vi "sorter.vi"() -> ()   [LabVIEW 2016]
uses:
  <vilib>/vision/NI_Vision_Development_Module.lvlib
panel:
  out "motor":bool
  out "green no.":dbl
  out "red no.":dbl
  out "?":dbl(graph)
  out "Sensor":bool
  in  "STOP":bool
  in  "START":bool
  in  "Stop (F)":bool
  out "?":dbl
  out "?":dbl
  out "green":bool
  out "red":bool
  out "?":dbl[](array[numeric]) format="%.2f"
  out "?":T1(plugin-control)
  # "Color Sorting Machine"
  # "Image Processing Indicators"
  # "Supervisory Control Panel"
  # "Motor Speed"
  # "Program Stop"
  # "Lamees Haitham El-Bakr\n             Supervisor \n         Dr : Ramy Farid"
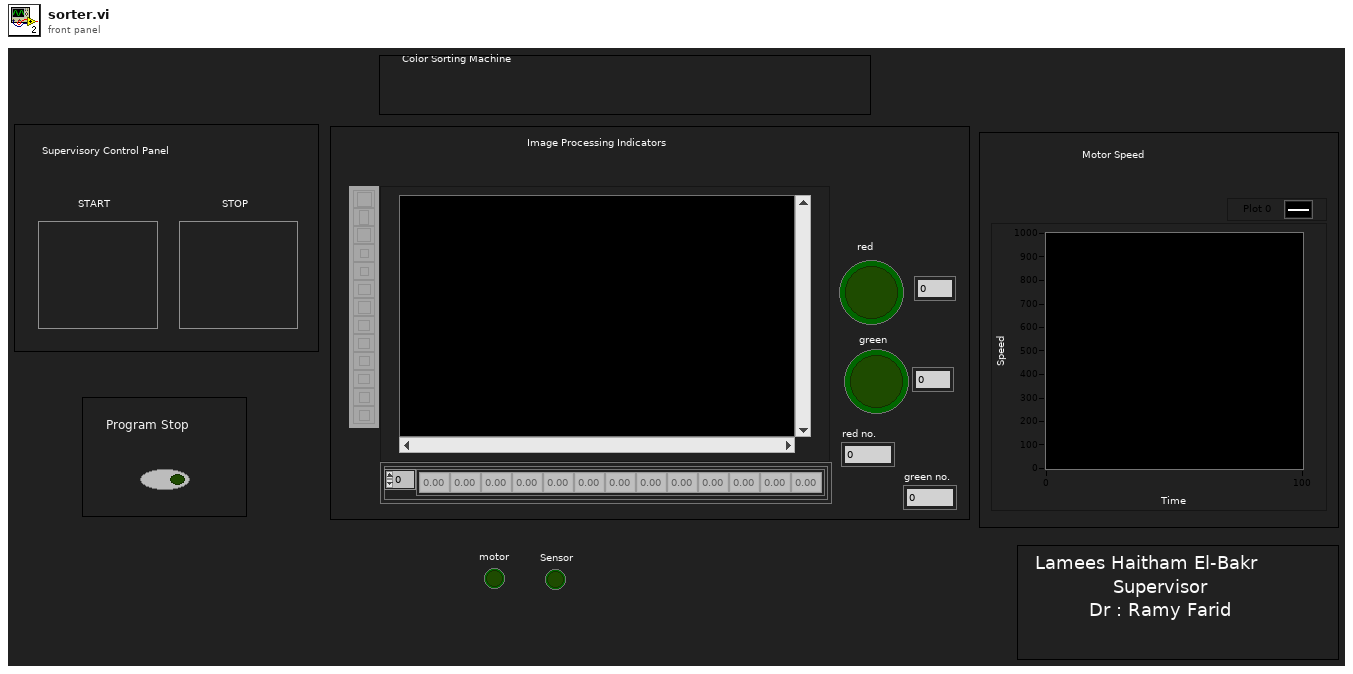
[diagram p1: front panel]
types:
  T1 = typedef "IMAQ Image.ctl" = refnum<image>
  T2 = enum16{"Read", "Write", "ReadWrite", "BufferedRead", "BufferedReadWrite"}
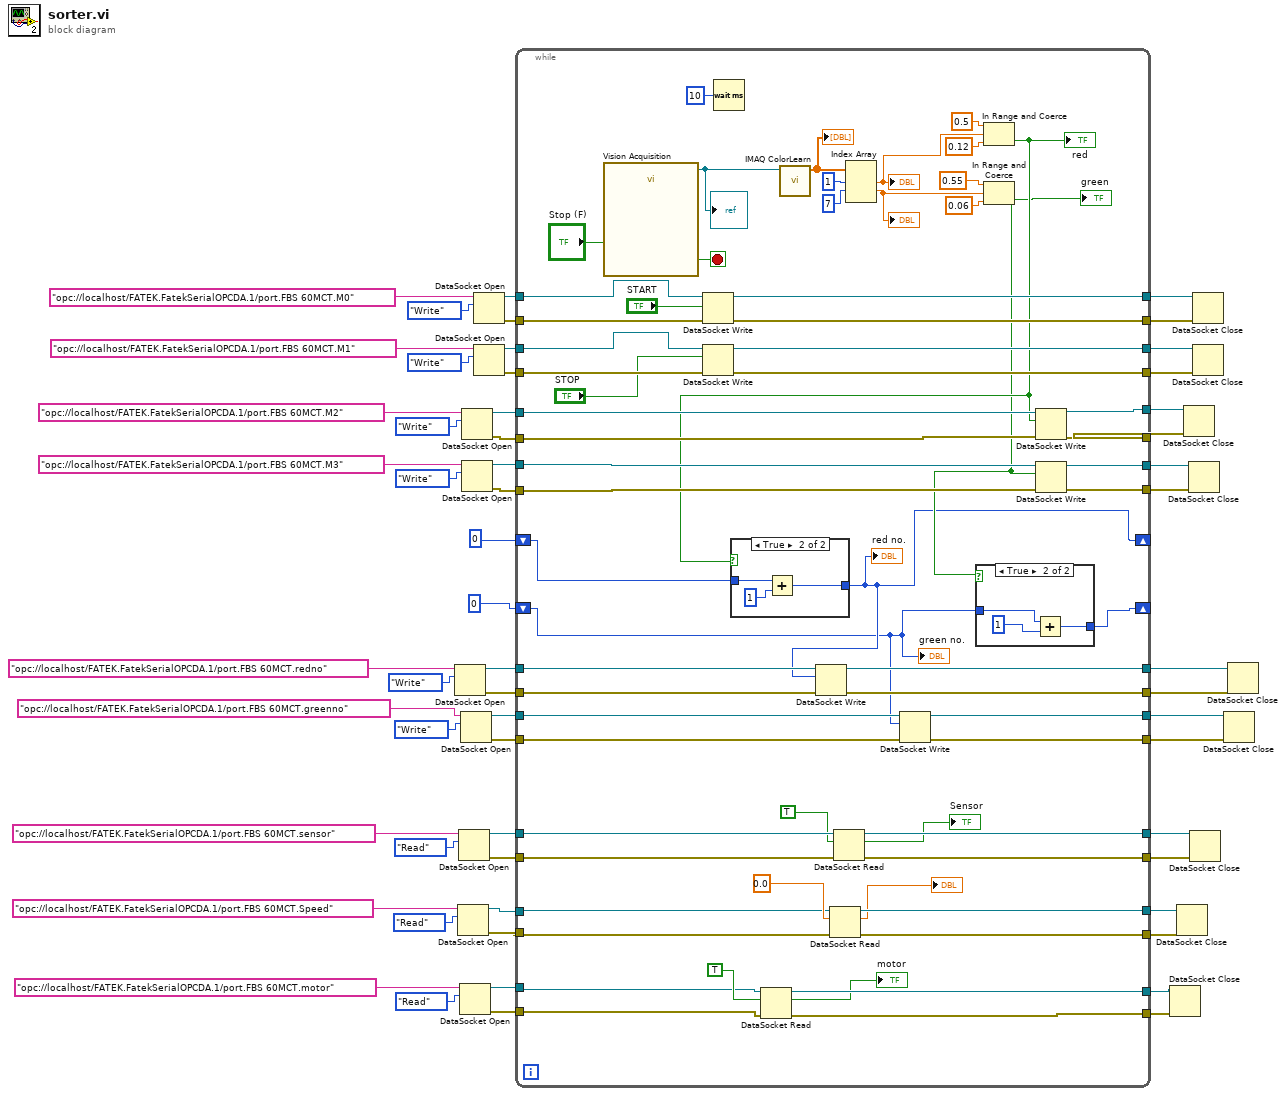
[diagram p0: block diagram]
diagram:
  n1 = DataSocket Open(10:T2."Write" ("mode"), 11:"opc://localhost/FATEK.FatekSerialOPCDA.1/port.FBS 60MCT.redno") -> (0:w9:errorcluster, 3:w10:refnum<k13>)  [unwired: 2 in]
  n2 = DataSocket Open(10:T2."Read" ("mode"), 11:"opc://localhost/FATEK.FatekSerialOPCDA.1/port.FBS 60MCT.Speed") -> (0:w23:errorcluster, 3:w24:refnum<k13>)  [unwired: 2 in]
  n3 = DataSocket Open(10:T2."Read" ("mode"), 11:"opc://localhost/FATEK.FatekSerialOPCDA.1/port.FBS 60MCT.sensor") -> (0:w29:errorcluster, 3:w30:refnum<k13>)  [unwired: 2 in]
  n4 = DataSocket Open(10:T2."Read" ("mode"), 11:"opc://localhost/FATEK.FatekSerialOPCDA.1/port.FBS 60MCT.motor") -> (0:w17:errorcluster, 3:w18:refnum<k13>)  [unwired: 2 in]
  n5 = DataSocket Open(10:T2."Write" ("mode"), 11:"opc://localhost/FATEK.FatekSerialOPCDA.1/port.FBS 60MCT.greenno") -> (0:w4:errorcluster, 3:w3:refnum<k13>)  [unwired: 2 in]
  n6 = DataSocket Open(10:T2."Write" ("mode"), 11:"opc://localhost/FATEK.FatekSerialOPCDA.1/port.FBS 60MCT.M2") -> (0:w39:errorcluster, 3:w40:refnum<k13>)  [unwired: 2 in]
  n7 = DataSocket Open(10:T2."Write" ("mode"), 11:"opc://localhost/FATEK.FatekSerialOPCDA.1/port.FBS 60MCT.M3") -> (0:w37:errorcluster, 3:w38:refnum<k13>)  [unwired: 2 in]
  n8 = DataSocket Open(10:T2."Write" ("mode"), 11:"opc://localhost/FATEK.FatekSerialOPCDA.1/port.FBS 60MCT.M0") -> (0:w51:errorcluster, 3:w52:refnum<k13>)  [unwired: 2 in]
  n9 = DataSocket Open(10:T2."Write" ("mode"), 11:"opc://localhost/FATEK.FatekSerialOPCDA.1/port.FBS 60MCT.M1") -> (0:w49:errorcluster, 3:w50:refnum<k13>)  [unwired: 2 in]
  n10 = while {
    tunnel: w52 -> [w107]
    tunnel: w51 -> [w106]
    tunnel: w50 -> [w105]
    tunnel: w49 -> [w104]
    tunnel: [w100] -> w48
    tunnel: [w103] -> w47
    tunnel: [w102] -> w46
    tunnel: [w101] -> w45
    tunnel: w40 -> [w99]
    tunnel: w39 -> [w98]
    tunnel: w38 -> [w97]
    tunnel: w37 -> [w96]
    tunnel: [w95] -> w36
    tunnel: [w94] -> w35
    tunnel: [w93] -> w34
    tunnel: [w92] -> w33
    tunnel: w30 -> [w89]
    tunnel: w29 -> [w88]
    tunnel: [w87] -> w28
    tunnel: [w86] -> w27
    tunnel: w24 -> [w82]
    tunnel: w23 -> [w81]
    tunnel: [w80] -> w22
    tunnel: [w79] -> w21
    tunnel: w18 -> [w76]
    tunnel: w17 -> [w75]
    tunnel: [w74] -> w16
    tunnel: [w73] -> w15
    shift-right: [w60] -> _
    shift-left: 0 -> [w70]
    shift-right: [w69] -> _
    shift-left: 0 -> [w59]
    tunnel: w10 -> [w68]
    tunnel: w9 -> [w67]
    tunnel: [w66] -> w8
    tunnel: [w65] -> w7
    tunnel: [w64] -> w6
    tunnel: [w63] -> w5
    tunnel: w4 -> [w62]
    tunnel: w3 -> [w61]
    stop <- w108 stop-if-true
    n11 = call "Vision Acquisition"("Stop (F)"="Stop (F)") -> ("Image Out"=w109:T1, "Stopped"=w108:bool)  [unwired: 24 in, 1 out]
    "?" <- w109
    n12 = DataSocket Write(8:w106, 10:"START", 11:w107) -> (0:w103:errorcluster, 3:w100:refnum<k13>)  [unwired: 1 in, 1 out]
    n13 = DataSocket Write(8:w104, 10:"STOP", 11:w105) -> (0:w101:errorcluster, 3:w102:refnum<k13>)  [unwired: 1 in, 1 out]
    n14 = Wait (ms)(milliseconds to wait=u32 10) -> ()  [unwired: 1 out]
    n15 = DataSocket Read(8:w75, 10:TRUE, 11:w76) -> (0:w73:errorcluster, 2:→"motor":bool, 3:w74:refnum<k13>)  [unwired: 2 in, 4 out]
    n16 = call "IMAQ ColorLearn"("Image"=w109) -> ("Color Spectrum"=w119:dbl[])  [unwired: 7 in, 1 out]
    "?" <- w119
    n17 = DataSocket Read(8:w81, 10:0.0, 11:w82) -> (0:w79:errorcluster, 2:→"?":dbl, 3:w80:refnum<k13>)  [unwired: 2 in, 4 out]
    n18 = DataSocket Read(8:w88, 10:TRUE, 11:w89) -> (0:w86:errorcluster, 2:→"Sensor":bool, 3:w87:refnum<k13>)  [unwired: 2 in, 4 out]
    n19 = Index Array(array=w119, index #1=1 ("index"), index #2=7 ("index")) -> (element #1=w112:dbl, element #2=w111:dbl)  [unwired: 1 in, 1 out]
    "?" <- w111
    "?" <- w112
    n20 = DataSocket Write(8:w62, 10:w59, 11:w61) -> (0:w63:errorcluster, 3:w64:refnum<k13>)  [unwired: 1 in, 1 out]
    n21 = In Range and Coerce(upper limit=0.5, x=w112, lower limit=0.12) -> (In Range?=w72:bool)  [unwired: 1 out]
    "red" <- w72
    n22 = case shown="True" w72 {
      tunnel: w70 -> [w120 w123]
      tunnel: [w120 w122] -> w60
      frame False {
      }
      frame True {
        n23 = Add(x=w123, y=1) -> (x+y=w122:i32)
      }
    }
    "red no." <- w60
    n24 = DataSocket Write(8:w67, 10:w60, 11:w68) -> (0:w65:errorcluster, 3:w66:refnum<k13>)  [unwired: 1 in, 1 out]
    n25 = In Range and Coerce(upper limit=0.55, x=w111, lower limit=0.06) -> (In Range?=w71:bool)  [unwired: 1 out]
    "green" <- w71
    n26 = case shown="True" w71 {
      tunnel: [w124 w127] -> w69
      tunnel: w59 -> [w124 w126]
      frame False {
      }
      frame True {
        n27 = Add(x=w126, y=1) -> (x+y=w127:i32)
      }
    }
    n28 = DataSocket Write(8:w98, 10:w72, 11:w99) -> (0:w94:errorcluster, 3:w95:refnum<k13>)  [unwired: 1 in, 1 out]
    n29 = DataSocket Write(8:w96, 10:w71, 11:w97) -> (0:w92:errorcluster, 3:w93:refnum<k13>)  [unwired: 1 in, 1 out]
    "green no." <- w59
  }
  n30 = DataSocket Close(8:w15, 11:w16) -> ()  [unwired: 1 in, 2 out]
  n31 = DataSocket Close(8:w21, 11:w22) -> ()  [unwired: 1 in, 2 out]
  n32 = DataSocket Close(8:w35, 11:w36) -> ()  [unwired: 1 in, 2 out]
  n33 = DataSocket Close(8:w33, 11:w34) -> ()  [unwired: 1 in, 2 out]
  n34 = DataSocket Close(8:w27, 11:w28) -> ()  [unwired: 1 in, 2 out]
  n35 = DataSocket Close(8:w47, 11:w48) -> ()  [unwired: 1 in, 2 out]
  n36 = DataSocket Close(8:w45, 11:w46) -> ()  [unwired: 1 in, 2 out]
  n37 = DataSocket Close(8:w5, 11:w6) -> ()  [unwired: 1 in, 2 out]
  n38 = DataSocket Close(8:w7, 11:w8) -> ()  [unwired: 1 in, 2 out]
